vi "WaveformComponent, Append Trailing Edge.vi"(0 "waveform in":waveform(dbl)={"t0"=timestamp(3474820848.0780005 s since 1904-01-01), "dt"=nan, "Y"=[]}, 1 "append parameters":T1={"offset"=0.5, "amplitude"=-2.0, "delay"=0.00019999999999999998, "leading edge"=0.0005, "pulse width"=0.0006, "trailing edge"=0.0005, "ref level %"=1.0} {"ref level %" format="%.3f"; "offset" format="%.3f"; "pulse width" format="%.1f"; "trailing edge" format="%.1f"; "amplitude" format="%.3f"; "delay" format="%.1f"; "leading edge" format="%.1f"}) -> (3 "waveform out":waveform(dbl)={"t0"=timestamp(-9593225999.921999 s since 1904-01-01), "dt"=nan, "Y"=[]})   [LabVIEW 2010]
uses:
  Pulse Parameters.ctl
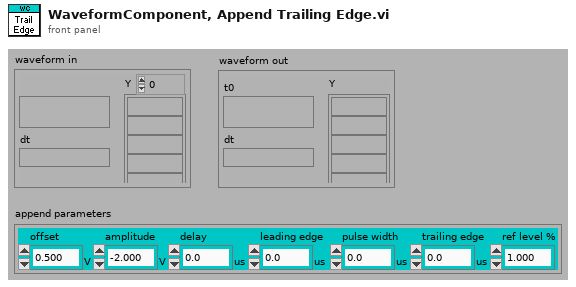
[diagram p1: front panel]
types:
  T1 = typedef "Pulse Parameters.ctl" = cluster{"offset":dbl[unit], "amplitude":dbl[unit], "delay":dbl[unit], "leading edge":dbl[unit], "pulse width":dbl[unit], "trailing edge":dbl[unit], "ref level %":dbl}
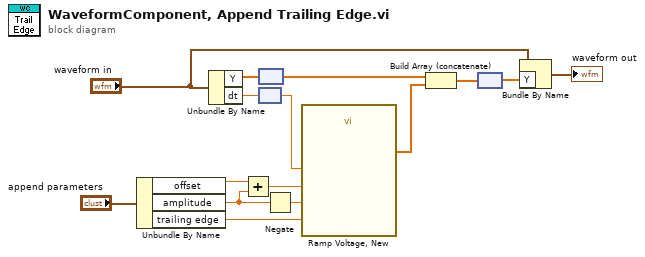
[diagram p0: block diagram]
diagram:
  n1 = Unbundle By Name("append parameters") -> ("offset"=w1:dbl[unit], "amplitude"=w2:dbl[unit], "trailing edge"=w13:dbl[unit])
  n2 = Unbundle By Name("waveform in") -> ("Y"=w11:dbl[], "dt"=w9:dbl)
  n3 = Add(x=w1, y=w2) -> (x+y=w3:dbl[unit])
  n4 = node(w11) -> (w7:dbl[unit][])
  n5 = node(w9) -> (w8:dbl[unit])
  n6 = Negate(x=w2) -> (-x=w4:dbl[unit])
  n7 = call "Ramp Voltage, New.vi"("offset (0.0)"=w3, "amplitude (0.0)"=w4, "dt"=w8, "total time"=w13) -> ("ramp"=w14:dbl[unit][])  [unwired: 1 in]
  n8 = Build Array (concatenate)(w7, w14) -> (w6:dbl[unit][])
  n9 = node(w6) -> (w15:dbl[])
  n10 = Bundle By Name(cluster="waveform in", "Y"=w15) -> (→"waveform out":waveform(dbl))
